vi "displacementSerialTest.vi"() -> ()   [LabVIEW 2016]
uses:
  <vilib>/Instr/_visa.llb/VISA Configure Serial Port (Instr).vi
panel:
  in  "SendMany":bool
  out "Time (us)":u32
  out "Response":string
  in  "Send":bool
  in  "Command":string
  in  "Stop":bool
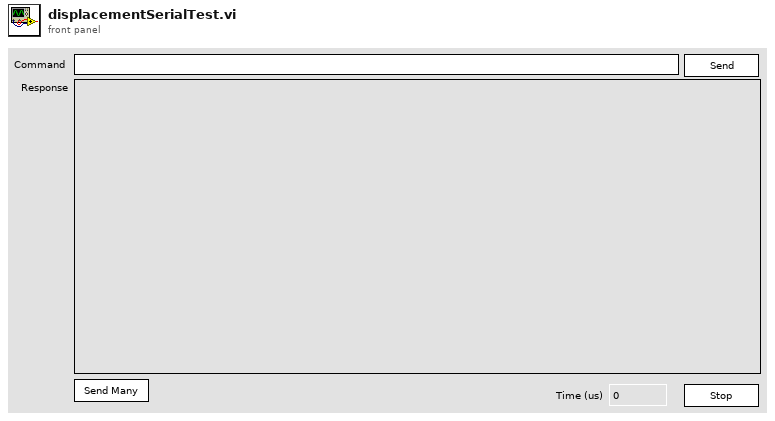
[diagram p1: front panel]
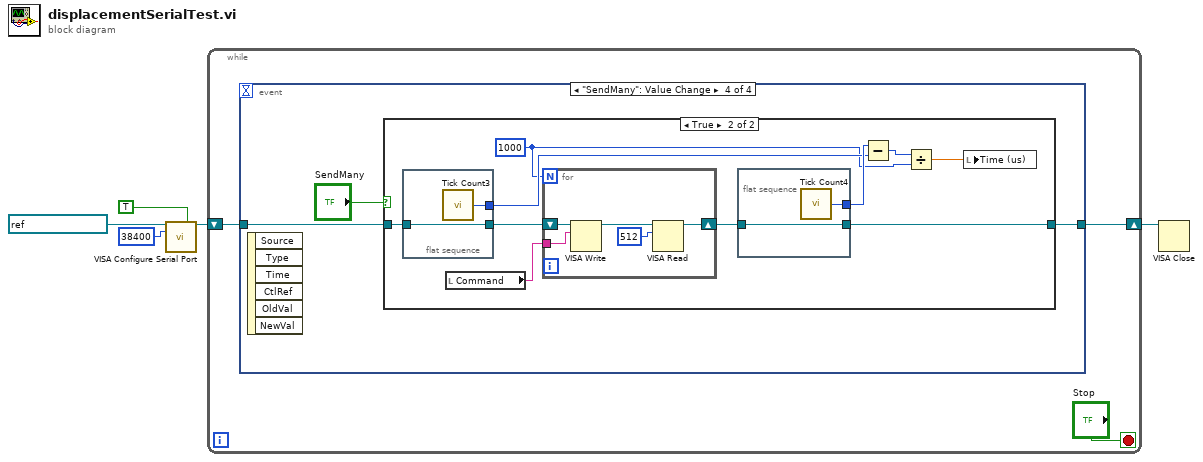
[diagram p0: block diagram]
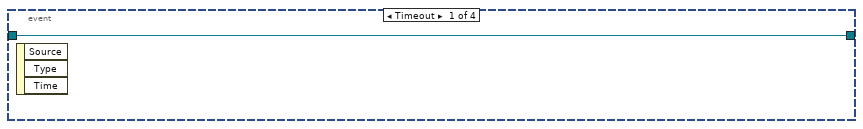
[diagram p2: hidden frame]
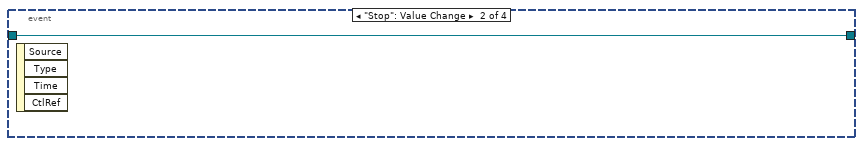
[diagram p3: hidden frame]
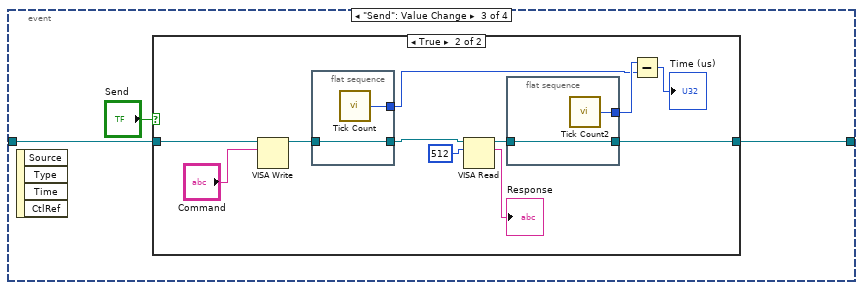
[diagram p4: hidden frame]
diagram:
  n1 = call-poly "VISA Configure Serial Port"("VISA resource name"=refnum<visa-resource-name> "ASRL1::INSTR", "Enable Termination\nChar (T)"=TRUE ("Enable Termination\nChar (T)"), "baud rate (9600)"=u32 38400) -> ("VISA resource name out"=w2:refnum<visa-resource-name>)  [unwired: 11 in, 1 out]
  n2 = while {
    shift-right: [w6] -> w1
    shift-left: w2 -> [w7]
    stop <- "Stop" stop-if-true
    n3 = event shown="[3] \"SendMany\": Value Change" {
      selector: _ -> [_ _ _ _]
      dyn-events: _ -> [_ _ _ _]
      timeout: _ -> [_ _ _ _]
      tunnel: w7 -> [w9 w10 w12 w31]
      tunnel: [w9 w10 w11 w30] -> w6
      event Timeout {
        n4 = event-data() -> ()  [unwired: 1 in, 3 out]
      }
      event "Stop": Value Change {
        n5 = event-data() -> ()  [unwired: 1 in, 4 out]
      }
      event "Send": Value Change {
        n6 = event-data() -> ()  [unwired: 1 in, 4 out]
        n7 = case shown="True" "Send" {
          tunnel: w12 -> [w14 w25]
          tunnel: [w14 w18] -> w11
          frame False {
          }
          frame True {
            n8 = VISA Write(VISA resource name=w25, write buffer="Command") -> (VISA resource name out=w21:refnum<visa-resource-name>)  [unwired: 1 in, 2 out]
            n9 = flat-sequence {
              tunnel: w21 -> [w29]
              tunnel: [w29] -> w20
              tunnel: [w28] -> w16
              frame #0 {
                n10 = call "Tick Count"() -> ("Tick Count(uSec)"=w28:u32)
              }
            }
            n11 = VISA Read(VISA resource name=w20, byte count=u32 512) -> (VISA resource name out=w19:refnum<visa-resource-name>, read buffer=→"Response":string)  [unwired: 1 in, 2 out]
            n12 = flat-sequence {
              tunnel: w19 -> [w27]
              tunnel: [w27] -> w18
              tunnel: [w26] -> w17
              frame #0 {
                n13 = call "Tick Count2"() -> ("Tick Count(uSec)"=w26:u32)
              }
            }
            n14 = Subtract(x=w17, y=w16) -> (x-y=→"Time (us)":u32)
          }
        }
      }
      event "SendMany": Value Change {
        n15 = event-data() -> ()  [unwired: 1 in, 6 out]
        n16 = case shown="True" "SendMany" {
          tunnel: w31 -> [w33 w43]
          tunnel: [w33 w40] -> w30
          frame False {
          }
          frame True {
            w35 = 1000
            n17 = flat-sequence {
              tunnel: w43 -> [w47]
              tunnel: [w47] -> w42
              tunnel: [w46] -> w38
              frame #0 {
                n18 = call "Tick Count3"() -> ("Tick Count(uSec)"=w46:u32)
              }
            }
            n19 = local read "Command"() -> (w37:string)
            n20 = for {
              N: w35 -> [_]
              shift-right: [w48] -> w41
              shift-left: w42 -> [w52]
              tunnel: w37 -> [w51]
              n21 = VISA Write(VISA resource name=w52, write buffer=w51) -> (VISA resource name out=w49:refnum<visa-resource-name>)  [unwired: 1 in, 2 out]
              n22 = VISA Read(VISA resource name=w49, byte count=u32 512) -> (VISA resource name out=w48:refnum<visa-resource-name>)  [unwired: 1 in, 3 out]
            }
            n23 = flat-sequence {
              tunnel: w41 -> [w45]
              tunnel: [w45] -> w40
              tunnel: [w44] -> w39
              frame #0 {
                n24 = call "Tick Count4"() -> ("Tick Count(uSec)"=w44:u32)
              }
            }
            n25 = Subtract(x=w39, y=w38) -> (x-y=w36:u32)
            n26 = Divide(x=w36, y=w35) -> (x/y=w34:dbl)
            n27 = local write "Time (us)"(w34) -> ()
          }
        }
      }
    }
  }
  n28 = VISA Close(VISA resource name=w1) -> ()  [unwired: 1 in, 1 out]
